vi "Autonomous Independent.vi"() -> ()   [LabVIEW 2013]
doc: "This VI is called when autonomous begins, and will automatically be terminated when autonomous ends. You can carry out timed or sensor driven robot movement independently without needing to return to the caller."
uses:
  Program Files (x86)/National Instruments/LabVIEW 2013/examples/FRC/Vision/2014 Target Detection/TargetType.ctl
  Robot Global Data.vi
  <vilib>/Rock Robotics/WPI/RobotDrive/WPI_RobotDriveArcadeDrive_Standard(NoSaturation).vi
  <vilib>/Rock Robotics/WPI/RobotDrive/WPI_RobotDriveGetSetRefNum.vi
  <vilib>/Rock Robotics/WPI/Joystick/WPI_JoystickGetSetRefNum.vi
panel:
  out "Distances":T2(array[cluster])
  out "[0].Distance (ft)":dbl
  out "Current Movement, for debugging":T3 {"Y Joystick Value" scale=1.0..-1.0; "X Joystick Value" scale=-1.0..1.0}
  in  "Array of robot movements":T4(array[cluster]) {"Y Joystick Value" scale=1.0..-1.0; "X Joystick Value" scale=-1.0..1.0}
  # "Be sure to right-click and choose Data Operations>>Make Current Value default if you want to save the array values with the VI"
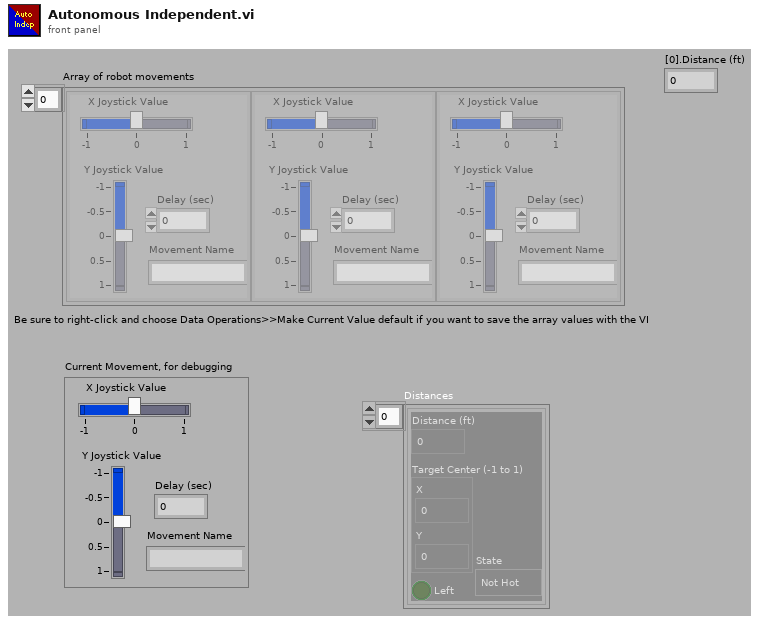
[diagram p1: front panel]
types:
  T1 = typedef "TargetType.ctl" = enum16{"Not Hot", "Hot"}
  T2 = cluster{"Distance (ft)":dbl, "Target Center (-1 to 1)":cluster{"X":dbl, "Y":dbl}, "Left":bool, "State":T1}[]
  T3 = cluster{"X Joystick Value":dbl, "Y Joystick Value":dbl, "Delay (sec)":dbl, "Movement Name":string}
  T4 = cluster{"X Joystick Value":dbl, "Y Joystick Value":dbl, "Delay (sec)":dbl, "Movement Name":string}[]
  T5 = typedef "WPI_JoystickDevRef.ctl" = cluster{"Device":T6}
  T6 = typedef "WPI_JoystickDeviceEnum.ctl" = enum16{"USB 1", "USB 2", "USB 3", "USB 4", "Kinect 1", "Kinect 2"}
  T7 = cluster{"axis 1 (x)":dbl, "axis 2 (y)":dbl, "axis 3 (throttle)":dbl, "axis 4":dbl, "axis 5":dbl, "axis 6":dbl}
  T8 = typedef "WPI_RobotDriveDevRef.ctl" = cluster{"DevStatus":errorcluster, "Motors[]":T9[], "Square Inputs":bool, "Max Output":dbl, "Isochronous":bool}
  T9 = typedef "WPI_MotorControlDeviceRef.ctl" = cluster{"DeviceStatus":errorcluster, "Type":enum16{"PWM", "CAN"}, "PWM":cluster{"Digital Module":T10, "PWM Channel":T11, "DeadBand":T12}, "CAN":cluster{"Device Number":u8, "Control Mode":T13, "Semaphore":T14, "Max Vout":dbl}, "Invert":bool, "TransformRef":T15, "InvTransformRef":T15}
  T10 = typedef "FPGA_TypedefDigitalModule.ctl" = enum16{"Digital Module 1", "Digital Module 2"}
  T11 = typedef "FPGA_DIOPWMChannel.ctl" = enum8{"PWM 1", "PWM 2", "PWM 3", "PWM 4", "PWM 5", "PWM 6", "PWM 7", "PWM 8", "PWM 9", "PWM 10", "Invalid"}
  T12 = typedef "WPI_PWMDeadband.ctl" = cluster{"Name":string, "maxPositivePwm":i32, "minPositivePwm":i32, "centerPwm":i32, "maxNegativePwm":i32, "minNegativePwm":i32, "angularRange":u16}
  T13 = typedef "WPI_CANJaguar_ControlMode.ctl" = enum8{"Percent VBus", "Current", "Speed", "Position", "Voltage"}
  T14 = typedef "Semaphore RefNum" = refnum<k1>
  T15 = typedef "WPI_PWMTransform_ConPane.ctl" = refnum<vi>
  T16 = cluster{"Distances[0]":cluster{"Distance (ft)":dbl, "Target Center (-1 to 1)":cluster{"X":dbl, "Y":dbl}, "Left":bool, "State":T1}, "Distances[1]":cluster{"Distance (ft)":dbl, "Target Center (-1 to 1)":cluster{"X":dbl, "Y":dbl}, "Left":bool, "State":T1}, "Distances[2]":cluster{"Distance (ft)":dbl, "Target Center (-1 to 1)":cluster{"X":dbl, "Y":dbl}, "Left":bool, "State":T1}, "Distances[3]":cluster{"Distance (ft)":dbl, "Target Center (-1 to 1)":cluster{"X":dbl, "Y":dbl}, "Left":bool, "State":T1}, "Distances[4]":cluster{"Distance (ft)":dbl, "Target Center (-1 to 1)":cluster{"X":dbl, "Y":dbl}, "Left":bool, "State":T1}, "Distances[5]":cluster{"Distance (ft)":dbl, "Target Center (-1 to 1)":cluster{"X":dbl, "Y":dbl}, "Left":bool, "State":T1}, "Distances[6]":cluster{"Distance (ft)":dbl, "Target Center (-1 to 1)":cluster{"X":dbl, "Y":dbl}, "Left":bool, "State":T1}, "Distances[7]":cluster{"Distance (ft)":dbl, "Target Center (-1 to 1)":cluster{"X":dbl, "Y":dbl}, "Left":bool, "State":T1}, "Distances[8]":cluster{"Distance (ft)":dbl, "Target Center (-1 to 1)":cluster{"X":dbl, "Y":dbl}, "Left":bool, "State":T1}}
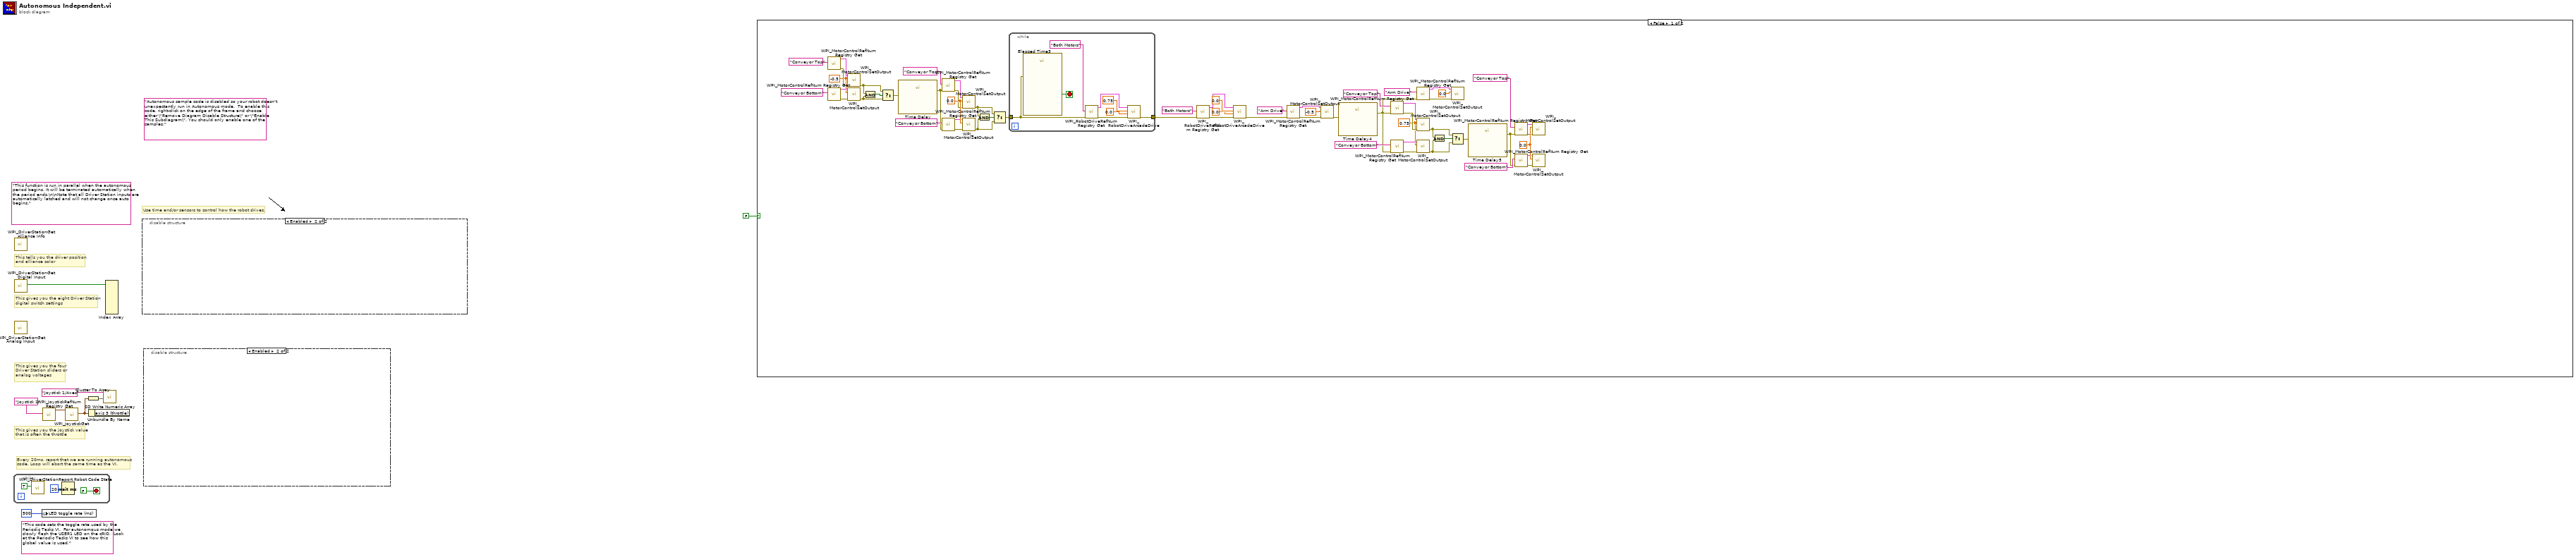
[diagram p0: block diagram]
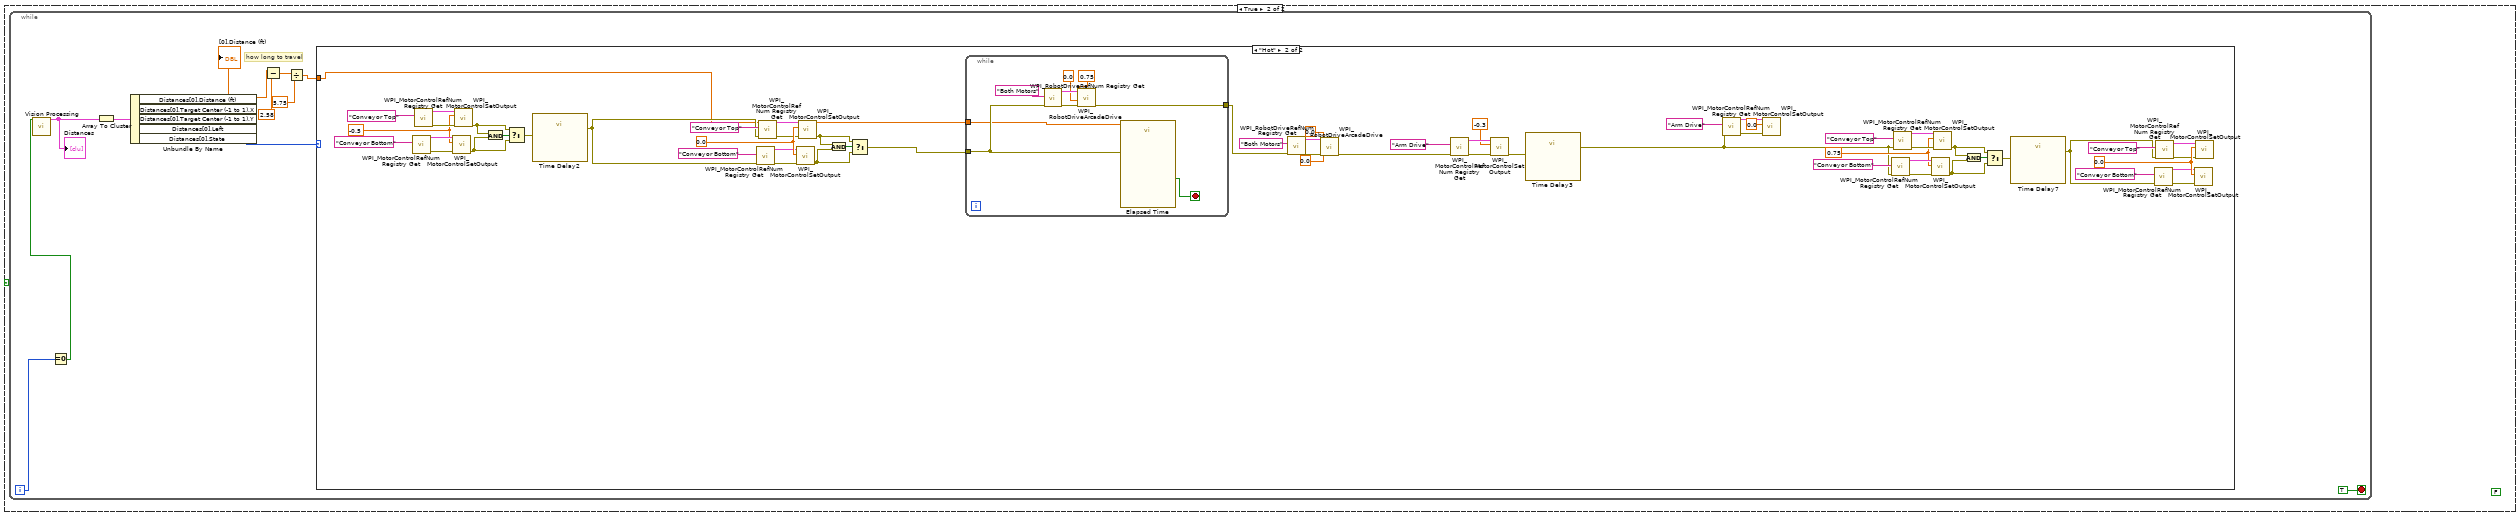
[diagram p2: hidden frame]
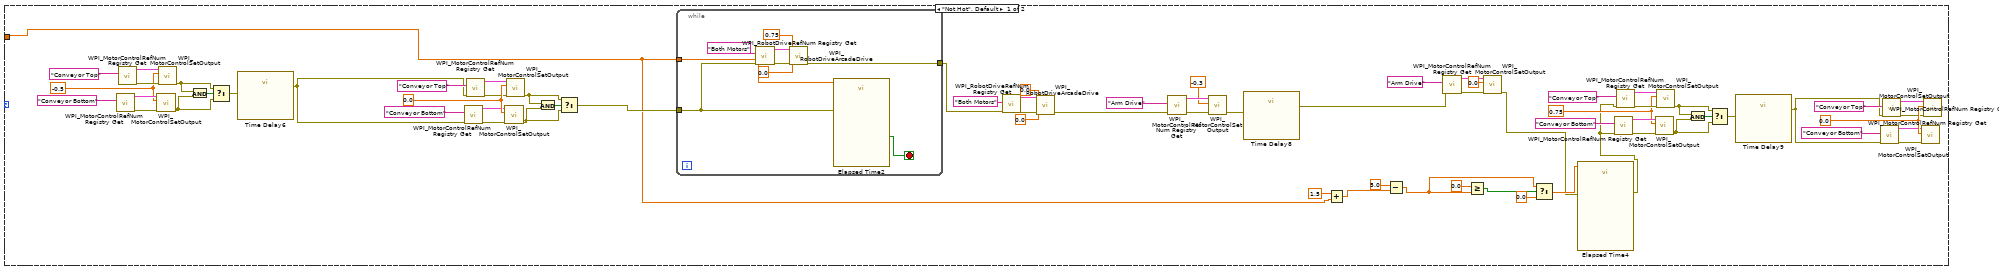
[diagram p3: hidden frame]
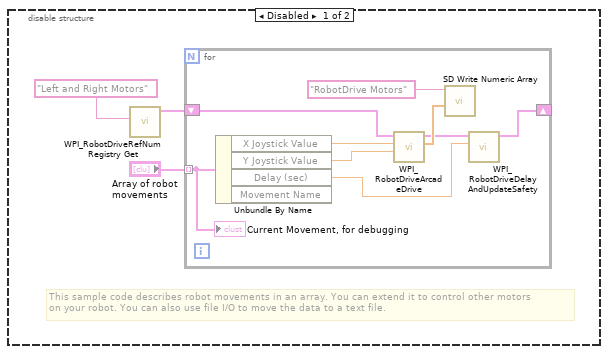
[diagram p4: hidden frame]
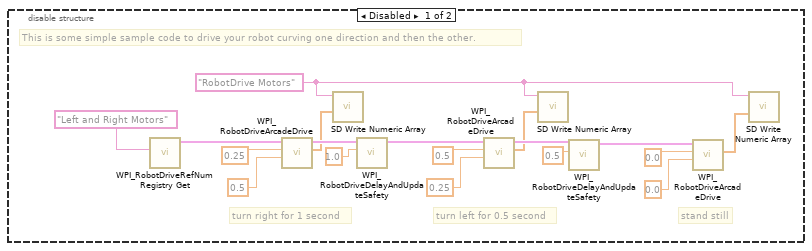
[diagram p5: hidden frame]
diagram:
  (unwired) "This code sets the toggle rate used by the Periodic Tasks VI.  For autonomous mode we slowly flash the USER1 LED on the cRIO.  Look at the Periodic Tasks VI to see how this global value is used."
  (unwired) "Autonomous sample code is disabled so your robot doesn't unexpectantly run in Autonomous mode.  To enable this code, right-click on the edge of the frame and choose either \"Remove Diagram Disable Structure\" or \"Enable This Subdiagram\". You should only enable one of the samples."
  (unwired) "This function is run in parallel when the autonomous period begins. It will be terminated automatically when the period ends.\n\nNote that all Driver Station inputs are automatically latched and will not change once auto begins."
  # "Every 20ms, report that we are running autonomous\ncode. Loop will abort the same time as the VI."
  # "This gives you the joystick value\nthat is often the throttle"
  # "Use time and/or sensors to control how the robot drives."
  # "This tells you the driver position\nand alliance color"
  # "This gives you the eight Driver Station\ndigital switch settings"
  # "This gives you the four\nDriver Station sliders or\nanalog voltages"
  n1 = while {
    stop <- FALSE stop-if-true
    n2 = call <vilib>:"WPI_DriverStationReport Robot Code State.vi"("Autonomous"=TRUE) -> ()  [unwired: 10 in, 1 out]
    n3 = Wait (ms)(milliseconds to wait=u32 20) -> ()  [unwired: 1 out]
  }
  n4 = call <vilib>:"WPI_DriverStationGet Alliance Info.vi"() -> ()  [unwired: 12 out]
  n5 = call <vilib>:"WPI_DriverStationGet Digital Input.vi"() -> ("Driver Station Digital Input (1-8)"=w8:bool[])  [unwired: 11 out]
  n6 = call <vilib>:"WPI_DriverStationGet Analog Input.vi"() -> ()  [unwired: 12 out]
  n7 = global write "Robot Global Data.vi" "LED toggle rate (ms)"(u32 500 ("LED ms toggle rate")) -> ()
  n8 = call <vilib>:"WPI_JoystickRefNum Registry Get.vi"("refnum name"="Joystick 1") -> ("JoystickDevRef"=w6:T5)  [unwired: 1 in, 9 out]
  n9 = call <vilib>:"WPI_JoystickGet.vi"("JoystickDevRef"=w6) -> ("Axes"=w3:T7)  [unwired: 1 in, 5 out]
  n10 = Cluster To Array(cluster=w3) -> (array=w4:dbl[])
  n11 = Unbundle By Name(w3) -> ()  [unwired: 1 out]
  n12 = call <vilib>:"SD Write Numeric Array.vi"("Numeric Array"=w4, "Name"="Joystick 1/Axes") -> ()  [unwired: 8 in, 2 out]
  n13 = Index Array(array=w8) -> ()  [unwired: 8 in, 8 out]
  n14 = disable-structure shown="Enabled" {
    frame Disabled {
      w12 = "RobotDrive Motors" ("Name")
      # "This is some simple sample code to drive your robot curving one direction and then the other."
      # "stand still"
      # "turn left for 0.5 second"
      # "turn right for 1 second"
      n15 = call <vilib>:"WPI_RobotDriveRefNum Registry Get.vi"("refnum name"="Left and Right Motors") -> ("RobotDriveDevRef"=w16:T8)  [unwired: 1 in, 9 out]
      n16 = call-poly <vilib>:"WPI_RobotDriveArcadeDrive.vi"("Y axis value"=0.5 ("X axis value"), "X axis value"=0.25, "RobotDriveDevRef"=w16) -> ("Motor Values"=w15:dbl[], "RobotDriveDevRef"=w23:T8)  [unwired: 1 in, 6 out]
      n17 = call <vilib>:"SD Write Numeric Array.vi"("Numeric Array"=w15, "Name"=w12) -> ()  [unwired: 8 in, 2 out]
      n18 = call <vilib>:"WPI_RobotDriveDelayAndUpdateSafety.vi"("Delay (s)"=1.0, "RobotDriveDevRef"=w23) -> ("RobotDriveDevRef 2"=w22:T8)  [unwired: 8 in, 1 out]
      n19 = call-poly <vilib>:"WPI_RobotDriveArcadeDrive.vi"("Y axis value"=0.25 ("X axis value"), "X axis value"=0.5, "RobotDriveDevRef"=w22) -> ("Motor Values"=w14:dbl[], "RobotDriveDevRef"=w21:T8)  [unwired: 1 in, 6 out]
      n20 = call <vilib>:"SD Write Numeric Array.vi"("Numeric Array"=w14, "Name"=w12) -> ()  [unwired: 8 in, 2 out]
      n21 = call <vilib>:"WPI_RobotDriveDelayAndUpdateSafety.vi"("Delay (s)"=0.5, "RobotDriveDevRef"=w21) -> ("RobotDriveDevRef 2"=w20:T8)  [unwired: 8 in, 1 out]
      n22 = call-poly <vilib>:"WPI_RobotDriveArcadeDrive.vi"("Y axis value"=0.0 ("X axis value"), "X axis value"=0.0, "RobotDriveDevRef"=w20) -> ("Motor Values"=w13:dbl[])  [unwired: 1 in, 7 out]
      n23 = call <vilib>:"SD Write Numeric Array.vi"("Numeric Array"=w13, "Name"=w12) -> ()  [unwired: 8 in, 2 out]
    }
    frame Enabled {
    }
  }
  n24 = disable-structure shown="Enabled" {
    frame Disabled {
      # "This sample code describes robot movements in an array. You can extend it to control other motors\non your robot. You can also use file I/O to move the data to a text file."
      n25 = call <vilib>:"WPI_RobotDriveRefNum Registry Get.vi"("refnum name"="Left and Right Motors") -> ("RobotDriveDevRef"=w31:T8)  [unwired: 1 in, 9 out]
      n26 = for {
        shift-right: [w37] -> _
        shift-left: w31 -> [w38]
        tunnel: "Array of robot movements" -> [w33] mode=indexing
        n27 = Unbundle By Name(w33) -> ("X Joystick Value"=w36:dbl, "Y Joystick Value"=w35:dbl, "Delay (sec)"=w34:dbl)  [unwired: 1 out]
        n28 = call-poly <vilib>:"WPI_RobotDriveArcadeDrive.vi"("Y axis value"=w35, "X axis value"=w36, "RobotDriveDevRef"=w38) -> ("Motor Values"=w40:dbl[], "RobotDriveDevRef"=w39:T8)  [unwired: 1 in, 6 out]
        n29 = call <vilib>:"SD Write Numeric Array.vi"("Numeric Array"=w40, "Name"="RobotDrive Motors") -> ()  [unwired: 8 in, 2 out]
        n30 = call <vilib>:"WPI_RobotDriveDelayAndUpdateSafety.vi"("Delay (s)"=w34, "RobotDriveDevRef"=w39) -> ("RobotDriveDevRef 2"=w37:T8)  [unwired: 8 in, 1 out]
        "Current Movement, for debugging" <- w33
      }
    }
    frame Enabled {
    }
  }
  n31 = case shown="False" FALSE {
    frame False {
      w60 = 0.0 ("Output")
      w72 = 0.75 ("Output")
      w86 = 0.0 ("Output")
      w94 = -0.5 ("Output")
      n32 = call <vilib>:"WPI_MotorControlRefNum Registry Get.vi"("refnum name"="Conveyor Top") -> ("error out"=w98:errorcluster, "MotorControlDevRef"=w99:T9)  [unwired: 9 in]
      n33 = call <vilib>:"WPI_MotorControlRefNum Registry Get.vi"("refnum name"="Conveyor Bottom") -> ("error out"=w97:errorcluster, "MotorControlDevRef"=w96:T9)  [unwired: 9 in]
      n34 = call <vilib>:"WPI_MotorControlSetOutput.vi"("error in (no error)"=w98, "Output"=w94, "MotorControlDevRef"=w99) -> ("error out"=w92:errorcluster)  [unwired: 6 in, 2 out]
      n35 = call <vilib>:"WPI_MotorControlSetOutput.vi"("error in (no error)"=w97, "Output"=w94, "MotorControlDevRef"=w96) -> ("error out"=w91:errorcluster)  [unwired: 6 in, 2 out]
      n36 = And(x=w92, y=w91) -> (x .and. y?=w93:bool)
      n37 = Select(t=w92, s=w93, f=w91) -> (s? t:f=w90:errorcluster)
      n38 = call "Time Delay"("error in (no error)"=w90) -> ("error out"=w79:errorcluster)  [unwired: 10 in]
      n39 = call <vilib>:"WPI_MotorControlRefNum Registry Get.vi"("error in (no error)"=w79, "refnum name"="Conveyor Top") -> ("error out"=w82:errorcluster, "MotorControlDevRef"=w81:T9)  [unwired: 8 in]
      n40 = call <vilib>:"WPI_MotorControlRefNum Registry Get.vi"("error in (no error)"=w79, "refnum name"="Conveyor Bottom") -> ("error out"=w83:errorcluster, "MotorControlDevRef"=w84:T9)  [unwired: 8 in]
      n41 = call <vilib>:"WPI_MotorControlSetOutput.vi"("error in (no error)"=w82, "Output"=w86, "MotorControlDevRef"=w81) -> ("error out"=w88:errorcluster)  [unwired: 6 in, 2 out]
      n42 = call <vilib>:"WPI_MotorControlSetOutput.vi"("error in (no error)"=w83, "Output"=w86, "MotorControlDevRef"=w84) -> ("error out"=w89:errorcluster)  [unwired: 6 in, 2 out]
      n43 = And(x=w88, y=w89) -> (x .and. y?=w87:bool)
      n44 = Select(t=w88, s=w87, f=w89) -> (s? t:f=w49:errorcluster)
      n45 = while {
        tunnel: w49 -> [w102]
        tunnel: [w101] -> w43
        stop <- w103 stop-if-true
        n46 = call "Elapsed Time3"("error in (no error)"=w102) -> ("Time has Elapsed"=w103:bool)  [unwired: 11 in, 7 out]
        n47 = call <vilib>:"WPI_RobotDriveRefNum Registry Get.vi"("error in (no error)"=w102, "refnum name"="Both Motors") -> ("error out"=w107:errorcluster, "RobotDriveDevRef"=w108:T8)  [unwired: 8 in]
        n48 = call-poly <vilib>:"WPI_RobotDriveArcadeDrive.vi"("error in (no error)"=w107, "Y axis value"=0.0, "X axis value"=0.75, "RobotDriveDevRef"=w108) -> ("error out"=w101:errorcluster)  [unwired: 5 in, 2 out]
      }
      n49 = call <vilib>:"WPI_RobotDriveRefNum Registry Get.vi"("error in (no error)"=w43, "refnum name"="Both Motors") -> ("error out"=w45:errorcluster, "RobotDriveDevRef"=w44:T8)  [unwired: 8 in]
      n50 = call-poly <vilib>:"WPI_RobotDriveArcadeDrive.vi"("error in (no error)"=w45, "Y axis value"=0.0, "X axis value"=0.0, "RobotDriveDevRef"=w44) -> ("error out"=w42:errorcluster)  [unwired: 5 in, 2 out]
      n51 = call <vilib>:"WPI_MotorControlRefNum Registry Get.vi"("error in (no error)"=w42, "refnum name"="Arm Drive") -> ("error out"=w68:errorcluster, "MotorControlDevRef"=w67:T9)  [unwired: 8 in]
      n52 = call <vilib>:"WPI_MotorControlSetOutput.vi"("error in (no error)"=w68, "Output"=-0.5 ("t"), "MotorControlDevRef"=w67) -> ("error out"=w65:errorcluster)  [unwired: 6 in, 2 out]
      n53 = call "Time Delay4"("error in (no error)"=w65) -> ("error out"=w50:errorcluster)  [unwired: 10 in]
      n54 = call <vilib>:"WPI_MotorControlRefNum Registry Get.vi"("error in (no error)"=w50, "refnum name"="Conveyor Top") -> ("error out"=w76:errorcluster, "MotorControlDevRef"=w77:T9)  [unwired: 8 in]
      n55 = call <vilib>:"WPI_MotorControlRefNum Registry Get.vi"("error in (no error)"=w50, "refnum name"="Conveyor Bottom") -> ("error out"=w75:errorcluster, "MotorControlDevRef"=w74:T9)  [unwired: 8 in]
      n56 = call <vilib>:"WPI_MotorControlRefNum Registry Get.vi"("error in (no error)"=w50, "refnum name"="Arm Drive") -> ("error out"=w62:errorcluster, "MotorControlDevRef"=w63:T9)  [unwired: 8 in]
      n57 = call <vilib>:"WPI_MotorControlSetOutput.vi"("error in (no error)"=w76, "Output"=w72, "MotorControlDevRef"=w77) -> ("error out"=w70:errorcluster)  [unwired: 6 in, 2 out]
      n58 = call <vilib>:"WPI_MotorControlSetOutput.vi"("error in (no error)"=w75, "Output"=w72, "MotorControlDevRef"=w74) -> ("error out"=w69:errorcluster)  [unwired: 6 in, 2 out]
      n59 = And(x=w70, y=w69) -> (x .and. y?=w71:bool)
      n60 = call <vilib>:"WPI_MotorControlSetOutput.vi"("error in (no error)"=w62, "Output"=0.0, "MotorControlDevRef"=w63) -> ()  [unwired: 6 in, 3 out]
      n61 = Select(t=w70, s=w71, f=w69) -> (s? t:f=w61:errorcluster)
      n62 = call "Time Delay5"("error in (no error)"=w61) -> ("error out"=w53:errorcluster)  [unwired: 10 in]
      n63 = call <vilib>:"WPI_MotorControlRefNum Registry Get.vi"("error in (no error)"=w53, "refnum name"="Conveyor Top") -> ("error out"=w56:errorcluster, "MotorControlDevRef"=w55:T9)  [unwired: 8 in]
      n64 = call <vilib>:"WPI_MotorControlRefNum Registry Get.vi"("error in (no error)"=w53, "refnum name"="Conveyor Bottom") -> ("error out"=w57:errorcluster, "MotorControlDevRef"=w58:T9)  [unwired: 8 in]
      n65 = call <vilib>:"WPI_MotorControlSetOutput.vi"("error in (no error)"=w56, "Output"=w60, "MotorControlDevRef"=w55) -> ()  [unwired: 6 in, 3 out]
      n66 = call <vilib>:"WPI_MotorControlSetOutput.vi"("error in (no error)"=w57, "Output"=w60, "MotorControlDevRef"=w58) -> ()  [unwired: 6 in, 3 out]
    }
    frame True {
      (unwired) FALSE
      n67 = while {
        i -> [w109]
        stop <- TRUE stop-if-true
        # "how long to travel"
        n68 = Equal To 0?(x=w109) -> (x = 0?=w110:bool)
        n69 = call "Vision Processing.vi"("Boolean"=w110) -> ("Distances"=w115:T2)  [unwired: 10 in]
        "Distances" <- w115
        n70 = Array To Cluster(array=w115) -> (cluster=w119:T16)
        n71 = Unbundle By Name(w119) -> ("Distances[0].Distance (ft)"=w117:dbl, "Distances[0].State"=w118:T1)  [unwired: 3 out]
        "[0].Distance (ft)" <- w117
        n72 = Subtract(x=w117, y=2.58) -> (x-y=w114:dbl)
        n73 = Divide(x=w114, y=5.75) -> (x/y=w112:dbl)
        n74 = case shown="\"Hot\"" w118 {
          tunnel: w112 -> [w129 w199]
          frame "Not Hot", Default {
            w139 = 0.0 ("Output")
            w144 = 0.75 ("Output")
            w176 = 0.0 ("Output")
            w183 = -0.5 ("Output")
            n75 = call <vilib>:"WPI_MotorControlRefNum Registry Get.vi"("refnum name"="Conveyor Bottom") -> ("error out"=w186:errorcluster, "MotorControlDevRef"=w185:T9)  [unwired: 9 in]
            n76 = call <vilib>:"WPI_MotorControlRefNum Registry Get.vi"("refnum name"="Conveyor Top") -> ("error out"=w187:errorcluster, "MotorControlDevRef"=w188:T9)  [unwired: 9 in]
            n77 = call <vilib>:"WPI_MotorControlSetOutput.vi"("error in (no error)"=w186, "Output"=w183, "MotorControlDevRef"=w185) -> ("error out"=w131:errorcluster)  [unwired: 6 in, 2 out]
            n78 = call <vilib>:"WPI_MotorControlSetOutput.vi"("error in (no error)"=w187, "Output"=w183, "MotorControlDevRef"=w188) -> ("error out"=w181:errorcluster)  [unwired: 6 in, 2 out]
            n79 = And(x=w181, y=w131) -> (x .and. y?=w182:bool)
            n80 = Select(t=w181, s=w182, f=w131) -> (s? t:f=w180:errorcluster)
            n81 = call "Time Delay6"("error in (no error)"=w180) -> ("error out"=w169:errorcluster)  [unwired: 10 in]
            n82 = call <vilib>:"WPI_MotorControlRefNum Registry Get.vi"("error in (no error)"=w169, "refnum name"="Conveyor Bottom") -> ("error out"=w173:errorcluster, "MotorControlDevRef"=w174:T9)  [unwired: 8 in]
            n83 = call <vilib>:"WPI_MotorControlRefNum Registry Get.vi"("error in (no error)"=w169, "refnum name"="Conveyor Top") -> ("error out"=w172:errorcluster, "MotorControlDevRef"=w171:T9)  [unwired: 8 in]
            n84 = call <vilib>:"WPI_MotorControlSetOutput.vi"("error in (no error)"=w173, "Output"=w176, "MotorControlDevRef"=w174) -> ("error out"=w179:errorcluster)  [unwired: 6 in, 2 out]
            n85 = call <vilib>:"WPI_MotorControlSetOutput.vi"("error in (no error)"=w172, "Output"=w176, "MotorControlDevRef"=w171) -> ("error out"=w178:errorcluster)  [unwired: 6 in, 2 out]
            n86 = And(x=w178, y=w179) -> (x .and. y?=w177:bool)
            n87 = Select(t=w178, s=w177, f=w179) -> (s? t:f=w158:errorcluster)
            n88 = while {
              tunnel: w158 -> [w194]
              tunnel: [w193] -> w152
              tunnel: w129 -> [w192]
              stop <- w195 stop-if-true
              n89 = call <vilib>:"WPI_RobotDriveRefNum Registry Get.vi"("error in (no error)"=w194, "refnum name"="Both Motors") -> ("error out"=w197:errorcluster, "RobotDriveDevRef"=w198:T8)  [unwired: 8 in]
              n90 = call-poly <vilib>:"WPI_RobotDriveArcadeDrive.vi"("error in (no error)"=w197, "Y axis value"=0.0, "X axis value"=0.75, "RobotDriveDevRef"=w198) -> ("error out"=w193:errorcluster)  [unwired: 5 in, 2 out]
              n91 = call "Elapsed Time2"("Time Target (s)"=w192, "error in (no error)"=w194) -> ("Time has Elapsed"=w195:bool)  [unwired: 10 in, 7 out]
            }
            n92 = call <vilib>:"WPI_RobotDriveRefNum Registry Get.vi"("error in (no error)"=w152, "refnum name"="Both Motors") -> ("error out"=w154:errorcluster, "RobotDriveDevRef"=w153:T8)  [unwired: 8 in]
            n93 = call-poly <vilib>:"WPI_RobotDriveArcadeDrive.vi"("error in (no error)"=w154, "Y axis value"=0.0, "X axis value"=0.0, "RobotDriveDevRef"=w153) -> ("error out"=w151:errorcluster)  [unwired: 5 in, 2 out]
            n94 = call <vilib>:"WPI_MotorControlRefNum Registry Get.vi"("error in (no error)"=w151, "refnum name"="Arm Drive") -> ("error out"=w168:errorcluster, "MotorControlDevRef"=w167:T9)  [unwired: 8 in]
            n95 = call <vilib>:"WPI_MotorControlSetOutput.vi"("error in (no error)"=w168, "Output"=-0.3 ("t"), "MotorControlDevRef"=w167) -> ("error out"=w165:errorcluster)  [unwired: 6 in, 2 out]
            n96 = call "Time Delay8"("error in (no error)"=w165) -> ("error out"=w159:errorcluster)  [unwired: 10 in]
            n97 = Add(x=1.5, y=w129) -> (x+y=w128:dbl)
            n98 = Subtract(x=5.0, y=w128) -> (x-y=w124:dbl)
            n99 = call <vilib>:"WPI_MotorControlRefNum Registry Get.vi"("error in (no error)"=w159, "refnum name"="Arm Drive") -> ("error out"=w162:errorcluster, "MotorControlDevRef"=w163:T9)  [unwired: 8 in]
            n100 = Greater Or Equal?(x=0.0, y=w124) -> (x >= y?=w125:bool)
            n101 = call <vilib>:"WPI_MotorControlSetOutput.vi"("error in (no error)"=w162, "Output"=0.0, "MotorControlDevRef"=w163) -> ("error out"=w120:errorcluster)  [unwired: 6 in, 2 out]
            n102 = Select(t=w124, s=w125, f=0.0) -> (s? t:f=w122:dbl)
            n103 = call "Elapsed Time4"("Time Target (s)"=w122, "error in (no error)"=w120) -> ("error out"=w121:errorcluster)  [unwired: 10 in, 7 out]
            n104 = call <vilib>:"WPI_MotorControlRefNum Registry Get.vi"("error in (no error)"=w121, "refnum name"="Conveyor Bottom") -> ("error out"=w147:errorcluster, "MotorControlDevRef"=w146:T9)  [unwired: 8 in]
            n105 = call <vilib>:"WPI_MotorControlRefNum Registry Get.vi"("error in (no error)"=w121, "refnum name"="Conveyor Top") -> ("error out"=w148:errorcluster, "MotorControlDevRef"=w149:T9)  [unwired: 8 in]
            n106 = call <vilib>:"WPI_MotorControlSetOutput.vi"("error in (no error)"=w147, "Output"=w144, "MotorControlDevRef"=w146) -> ("error out"=w141:errorcluster)  [unwired: 6 in, 2 out]
            n107 = call <vilib>:"WPI_MotorControlSetOutput.vi"("error in (no error)"=w148, "Output"=w144, "MotorControlDevRef"=w149) -> ("error out"=w142:errorcluster)  [unwired: 6 in, 2 out]
            n108 = And(x=w142, y=w141) -> (x .and. y?=w143:bool)
            n109 = Select(t=w142, s=w143, f=w141) -> (s? t:f=w140:errorcluster)
            n110 = call "Time Delay9"("error in (no error)"=w140) -> ("error out"=w132:errorcluster)  [unwired: 10 in]
            n111 = call <vilib>:"WPI_MotorControlRefNum Registry Get.vi"("error in (no error)"=w132, "refnum name"="Conveyor Bottom") -> ("error out"=w136:errorcluster, "MotorControlDevRef"=w137:T9)  [unwired: 8 in]
            n112 = call <vilib>:"WPI_MotorControlRefNum Registry Get.vi"("error in (no error)"=w132, "refnum name"="Conveyor Top") -> ("error out"=w135:errorcluster, "MotorControlDevRef"=w134:T9)  [unwired: 8 in]
            n113 = call <vilib>:"WPI_MotorControlSetOutput.vi"("error in (no error)"=w136, "Output"=w139, "MotorControlDevRef"=w137) -> ()  [unwired: 6 in, 3 out]
            n114 = call <vilib>:"WPI_MotorControlSetOutput.vi"("error in (no error)"=w135, "Output"=w139, "MotorControlDevRef"=w134) -> ()  [unwired: 6 in, 3 out]
          }
          frame "Hot" {
            w218 = 0.0 ("Output")
            w230 = 0.75 ("Output")
            w244 = 0.0 ("Output")
            w252 = -0.5 ("Output")
            n115 = call <vilib>:"WPI_MotorControlRefNum Registry Get.vi"("refnum name"="Conveyor Bottom") -> ("error out"=w255:errorcluster, "MotorControlDevRef"=w254:T9)  [unwired: 9 in]
            n116 = call <vilib>:"WPI_MotorControlRefNum Registry Get.vi"("refnum name"="Conveyor Top") -> ("error out"=w256:errorcluster, "MotorControlDevRef"=w257:T9)  [unwired: 9 in]
            n117 = call <vilib>:"WPI_MotorControlSetOutput.vi"("error in (no error)"=w255, "Output"=w252, "MotorControlDevRef"=w254) -> ("error out"=w249:errorcluster)  [unwired: 6 in, 2 out]
            n118 = call <vilib>:"WPI_MotorControlSetOutput.vi"("error in (no error)"=w256, "Output"=w252, "MotorControlDevRef"=w257) -> ("error out"=w250:errorcluster)  [unwired: 6 in, 2 out]
            n119 = And(x=w250, y=w249) -> (x .and. y?=w251:bool)
            n120 = Select(t=w250, s=w251, f=w249) -> (s? t:f=w248:errorcluster)
            n121 = call "Time Delay2"("error in (no error)"=w248) -> ("error out"=w237:errorcluster)  [unwired: 10 in]
            n122 = call <vilib>:"WPI_MotorControlRefNum Registry Get.vi"("error in (no error)"=w237, "refnum name"="Conveyor Bottom") -> ("error out"=w241:errorcluster, "MotorControlDevRef"=w242:T9)  [unwired: 8 in]
            n123 = call <vilib>:"WPI_MotorControlRefNum Registry Get.vi"("error in (no error)"=w237, "refnum name"="Conveyor Top") -> ("error out"=w240:errorcluster, "MotorControlDevRef"=w239:T9)  [unwired: 8 in]
            n124 = call <vilib>:"WPI_MotorControlSetOutput.vi"("error in (no error)"=w241, "Output"=w244, "MotorControlDevRef"=w242) -> ("error out"=w247:errorcluster)  [unwired: 6 in, 2 out]
            n125 = call <vilib>:"WPI_MotorControlSetOutput.vi"("error in (no error)"=w240, "Output"=w244, "MotorControlDevRef"=w239) -> ("error out"=w246:errorcluster)  [unwired: 6 in, 2 out]
            n126 = And(x=w246, y=w247) -> (x .and. y?=w245:bool)
            n127 = Select(t=w246, s=w245, f=w247) -> (s? t:f=w207:errorcluster)
            n128 = while {
              tunnel: w207 -> [w261]
              tunnel: [w260] -> w201
              tunnel: w199 -> [w259]
              stop <- w262 stop-if-true
              n129 = call <vilib>:"WPI_RobotDriveRefNum Registry Get.vi"("error in (no error)"=w261, "refnum name"="Both Motors") -> ("error out"=w266:errorcluster, "RobotDriveDevRef"=w267:T8)  [unwired: 8 in]
              n130 = call-poly <vilib>:"WPI_RobotDriveArcadeDrive.vi"("error in (no error)"=w266, "Y axis value"=0.0, "X axis value"=0.75, "RobotDriveDevRef"=w267) -> ("error out"=w260:errorcluster)  [unwired: 5 in, 2 out]
              n131 = call "Elapsed Time"("Time Target (s)"=w259, "error in (no error)"=w261) -> ("Time has Elapsed"=w262:bool)  [unwired: 10 in, 7 out]
            }
            n132 = call <vilib>:"WPI_RobotDriveRefNum Registry Get.vi"("error in (no error)"=w201, "refnum name"="Both Motors") -> ("error out"=w203:errorcluster, "RobotDriveDevRef"=w202:T8)  [unwired: 8 in]
            n133 = call-poly <vilib>:"WPI_RobotDriveArcadeDrive.vi"("error in (no error)"=w203, "Y axis value"=0.0, "X axis value"=0.0, "RobotDriveDevRef"=w202) -> ("error out"=w200:errorcluster)  [unwired: 5 in, 2 out]
            n134 = call <vilib>:"WPI_MotorControlRefNum Registry Get.vi"("error in (no error)"=w200, "refnum name"="Arm Drive") -> ("error out"=w226:errorcluster, "MotorControlDevRef"=w225:T9)  [unwired: 8 in]
            n135 = call <vilib>:"WPI_MotorControlSetOutput.vi"("error in (no error)"=w226, "Output"=-0.3 ("t"), "MotorControlDevRef"=w225) -> ("error out"=w223:errorcluster)  [unwired: 6 in, 2 out]
            n136 = call "Time Delay3"("error in (no error)"=w223) -> ("error out"=w208:errorcluster)  [unwired: 10 in]
            n137 = call <vilib>:"WPI_MotorControlRefNum Registry Get.vi"("error in (no error)"=w208, "refnum name"="Arm Drive") -> ("error out"=w220:errorcluster, "MotorControlDevRef"=w221:T9)  [unwired: 8 in]
            n138 = call <vilib>:"WPI_MotorControlSetOutput.vi"("error in (no error)"=w220, "Output"=0.0, "MotorControlDevRef"=w221) -> ()  [unwired: 6 in, 3 out]
            n139 = call <vilib>:"WPI_MotorControlRefNum Registry Get.vi"("error in (no error)"=w208, "refnum name"="Conveyor Bottom") -> ("error out"=w233:errorcluster, "MotorControlDevRef"=w232:T9)  [unwired: 8 in]
            n140 = call <vilib>:"WPI_MotorControlRefNum Registry Get.vi"("error in (no error)"=w208, "refnum name"="Conveyor Top") -> ("error out"=w234:errorcluster, "MotorControlDevRef"=w235:T9)  [unwired: 8 in]
            n141 = call <vilib>:"WPI_MotorControlSetOutput.vi"("error in (no error)"=w233, "Output"=w230, "MotorControlDevRef"=w232) -> ("error out"=w227:errorcluster)  [unwired: 6 in, 2 out]
            n142 = call <vilib>:"WPI_MotorControlSetOutput.vi"("error in (no error)"=w234, "Output"=w230, "MotorControlDevRef"=w235) -> ("error out"=w228:errorcluster)  [unwired: 6 in, 2 out]
            n143 = And(x=w228, y=w227) -> (x .and. y?=w229:bool)
            n144 = Select(t=w228, s=w229, f=w227) -> (s? t:f=w219:errorcluster)
            n145 = call "Time Delay7"("error in (no error)"=w219) -> ("error out"=w211:errorcluster)  [unwired: 10 in]
            n146 = call <vilib>:"WPI_MotorControlRefNum Registry Get.vi"("error in (no error)"=w211, "refnum name"="Conveyor Bottom") -> ("error out"=w215:errorcluster, "MotorControlDevRef"=w216:T9)  [unwired: 8 in]
            n147 = call <vilib>:"WPI_MotorControlRefNum Registry Get.vi"("error in (no error)"=w211, "refnum name"="Conveyor Top") -> ("error out"=w214:errorcluster, "MotorControlDevRef"=w213:T9)  [unwired: 8 in]
            n148 = call <vilib>:"WPI_MotorControlSetOutput.vi"("error in (no error)"=w215, "Output"=w218, "MotorControlDevRef"=w216) -> ()  [unwired: 6 in, 3 out]
            n149 = call <vilib>:"WPI_MotorControlSetOutput.vi"("error in (no error)"=w214, "Output"=w218, "MotorControlDevRef"=w213) -> ()  [unwired: 6 in, 3 out]
          }
        }
      }
    }
  }
